vi "tap_stim_rec_async_2.vi"(0 "Convert Power to Voltage B":bool, 2 "voltages/power B":dbl[](array[numeric]), 3 "SSH password":string, 4 "Transfer and Run Date Folder After Experiment":bool, 5 "SSH user name":string, 6 "Tags":string, 7 "Frames":i32, 8 "Convert Power to Voltage":bool, 9 "voltages/power A":dbl[](array[numeric]), 10 "parameters":string[](array[string]), 11 "parameters headers":string[](array[string])) -> ()   [LabVIEW 2014]
uses:
  <vilib>/vision/driver/IMAQdx.llb/IMAQdx Acquisition Mode.ctl
  <vilib>/userdefined/High Color/IMAQdx.ctl
  <vilib>/vision/driver/IMAQdx.llb/IMAQdx Buffer Number Mode.ctl
  <vilib>/Utility/file.llb/Write To Spreadsheet File (DBL).vi
  <vilib>/Utility/file.llb/Write To Spreadsheet File (string).vi
  <vilib>/Utility/file.llb/Read From Spreadsheet File (string).vi
  <vilib>/vision/driver/NI_Vision_Acquisition_Software.lvlib
panel:
  out "Current Voltage B":dbl
  out "Current Voltage A":dbl
  out "Saved Buffer Number":u32
  out "ProcessFrameRate":dbl
  out "# elements in queue":i32
  out "CameraFrameRate":dbl
  out "Camera Buffer Number":u32
  out "Image":T1(plugin-control)
  out "JPEG Quality":dbl
  out "Error":string
  out "Save Directory":path
  in  "stop":bool
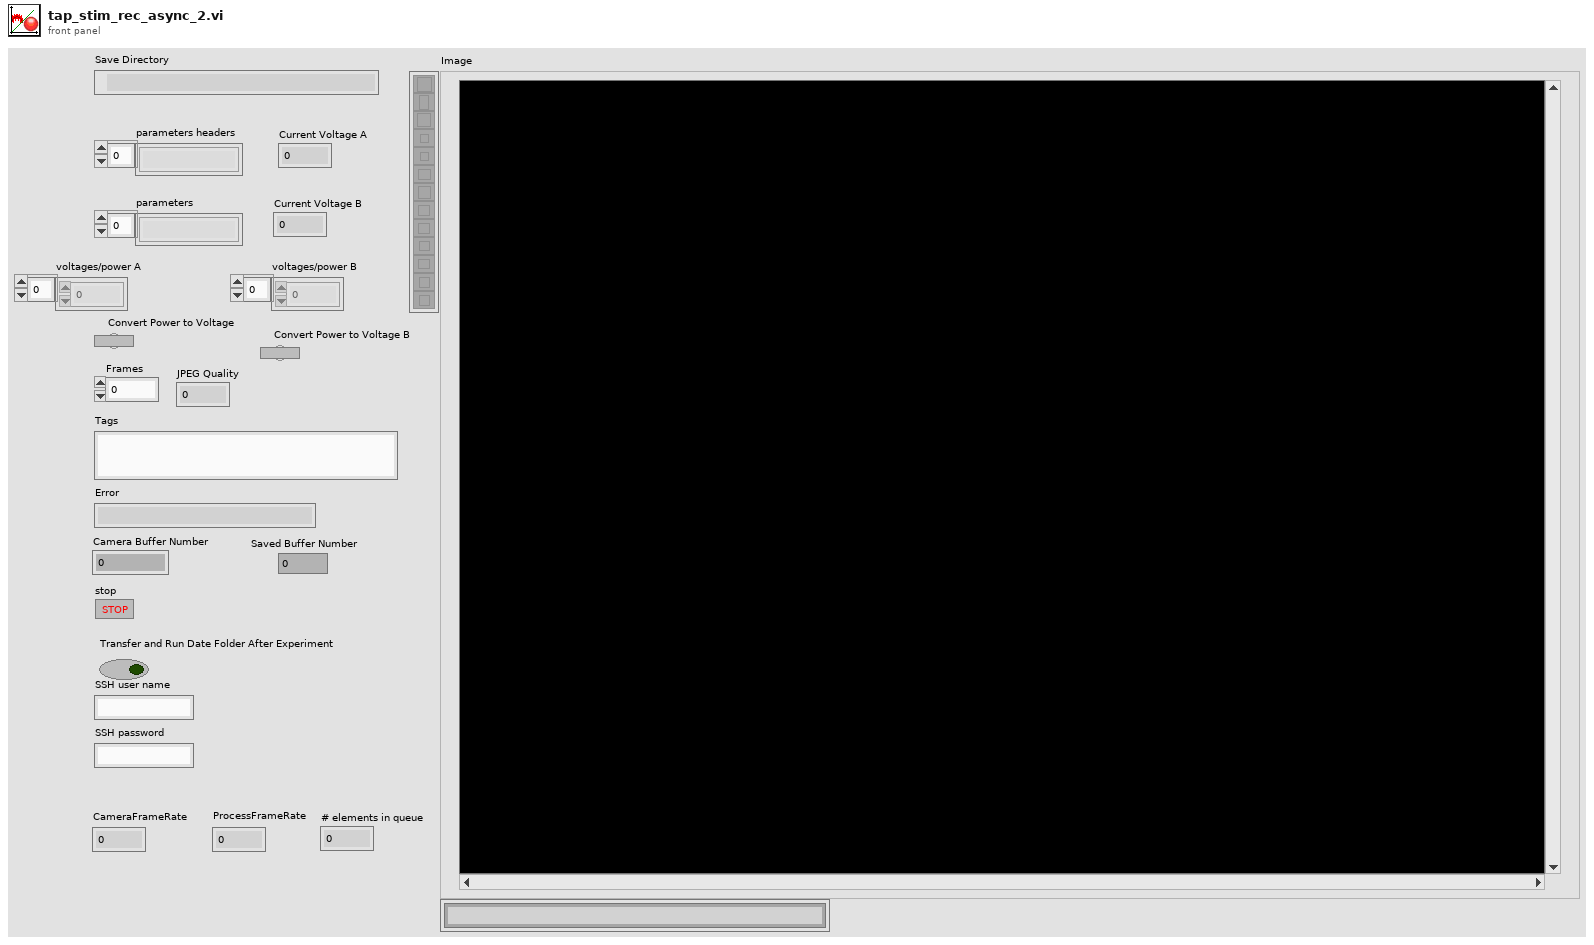
[diagram p1: front panel]
types:
  T1 = typedef "IMAQ Image.ctl" = refnum<image>
  T2 = typedef "IMAQdx.ctl" = refnum<k21>
  T3 = typedef "NI_Vision_Acquisition_Software.lvlib/IMAQdx Buffer Number Mode.ctl" = enum32{"Next", "Last", "Buffer Number"}
  T4 = typedef "Image Type" = u32
  T5 = typedef "NI_Vision_Acquisition_Software.lvlib/IMAQdx Acquisition Mode.ctl" = enum32{"One Shot", "Continuous"}
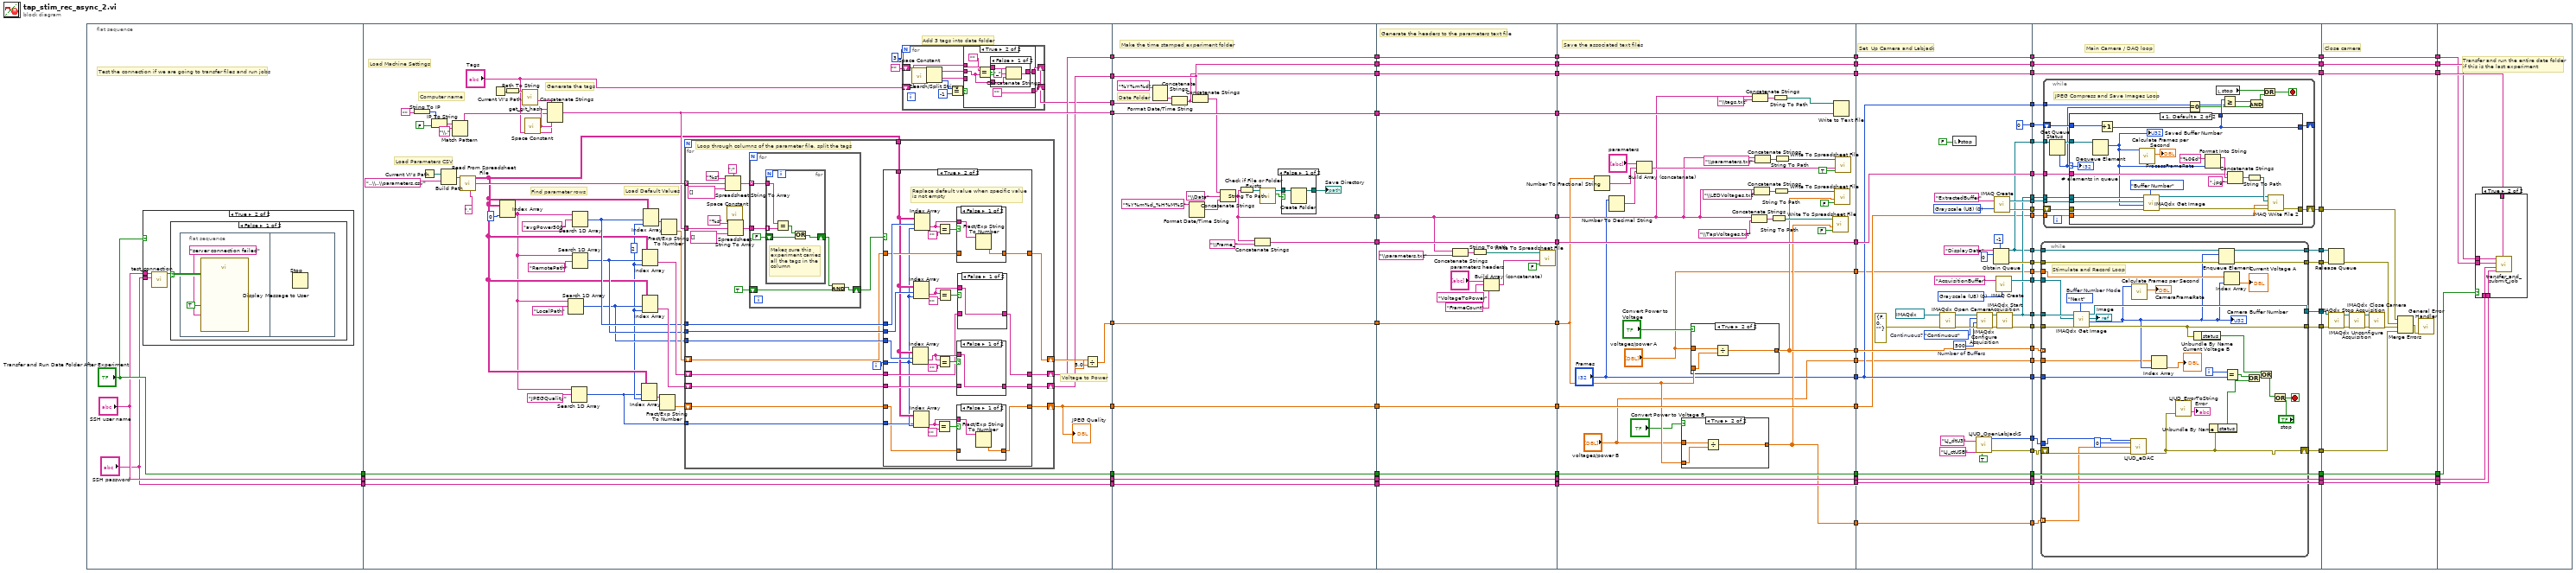
[diagram p0: block diagram]
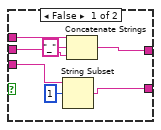
[diagram p4: hidden frame]
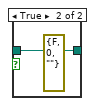
[diagram p11: hidden frame]
diagram:
  n1 = flat-sequence {
    tunnel: ["Transfer and Run Date Folder After Experiment"] -> w56
    tunnel: ["SSH user name"] -> w55
    tunnel: ["SSH password"] -> w54
    tunnel: [w138] -> w86
    tunnel: [w121] -> w85
    tunnel: [w112] -> w76
    tunnel: [w113] -> w75
    tunnel: w56 -> [w130]
    tunnel: w55 -> [w129]
    tunnel: w54 -> [w128]
    tunnel: [w130] -> w47
    tunnel: [w129] -> w40
    tunnel: [w128] -> w39
    tunnel: [w109] -> w32
    tunnel: [w100] -> w31
    tunnel: [w274] -> w70
    tunnel: [w273] -> w68
    tunnel: [w272] -> w66
    tunnel: [w271] -> w64
    tunnel: [w253] -> w62
    tunnel: [w255] -> w60
    tunnel: [w270] -> w58
    tunnel: w75 -> [w270]
    tunnel: w76 -> [w255]
    tunnel: w85 -> [w271]
    tunnel: w86 -> [w272]
    tunnel: [w262] -> w48
    tunnel: w47 -> [w262]
    tunnel: [w261] -> w41
    tunnel: w40 -> [w261]
    tunnel: w39 -> [w260]
    tunnel: [w260] -> w38
    tunnel: w32 -> [w256]
    tunnel: w31 -> [w252]
    tunnel: [w252] -> w28
    tunnel: w70 -> [w296]
    tunnel: [w296] -> w69
    tunnel: w68 -> [w282]
    tunnel: [w282] -> w67
    tunnel: w66 -> [w295]
    tunnel: [w295] -> w65
    tunnel: w64 -> [w294]
    tunnel: [w294] -> w63
    tunnel: w62 -> [w293]
    tunnel: [w293] -> w61
    tunnel: w60 -> [w292]
    tunnel: [w292] -> w59
    tunnel: w58 -> [w291]
    tunnel: [w291] -> w57
    tunnel: [w281] -> w49
    tunnel: w48 -> [w281]
    tunnel: [w280] -> w42
    tunnel: w41 -> [w280]
    tunnel: w38 -> [w279]
    tunnel: [w279] -> w37
    tunnel: [w278] -> w29
    tunnel: w28 -> [w278]
    tunnel: w69 -> [w331]
    tunnel: [w331] -> w91
    tunnel: [w301] -> w89
    tunnel: ["Frames"] -> w88
    tunnel: w67 -> [w302]
    tunnel: w65 -> [w308]
    tunnel: w63 -> [w311]
    tunnel: w61 -> [w320]
    tunnel: [w320] -> w81
    tunnel: [w319] -> w77
    tunnel: w59 -> [w319]
    tunnel: [w318] -> w71
    tunnel: w57 -> [w318]
    tunnel: [w314] -> w50
    tunnel: w49 -> [w314]
    tunnel: [w313] -> w43
    tunnel: w42 -> [w313]
    tunnel: w37 -> [w312]
    tunnel: [w312] -> w36
    tunnel: [w310] -> w30
    tunnel: w29 -> [w310]
    tunnel: [w300] -> w7
    tunnel: ["voltages/power A"] -> w6
    tunnel: ["voltages/power B"] -> w4
    tunnel: w91 -> [w352]
    tunnel: [w380] -> w90
    tunnel: w89 -> [w380]
    tunnel: w88 -> [w351]
    tunnel: [w351] -> w87
    tunnel: [w379] -> w82
    tunnel: w81 -> [w379]
    tunnel: [w378] -> w78
    tunnel: w77 -> [w378]
    tunnel: [w377] -> w72
    tunnel: w71 -> [w377]
    tunnel: [w376] -> w51
    tunnel: w50 -> [w376]
    tunnel: [w375] -> w44
    tunnel: w43 -> [w375]
    tunnel: w36 -> [w374]
    tunnel: [w374] -> w35
    tunnel: w30 -> [w349]
    tunnel: [w358] -> w27
    tunnel: [w353] -> w26
    tunnel: [w357] -> w25
    tunnel: [w356] -> w24
    tunnel: [w350] -> w23
    tunnel: [w355] -> w20
    tunnel: [w354] -> w19
    tunnel: [w353] -> w18
    tunnel: [w352] -> w17
    tunnel: [w351] -> w16
    tunnel: [w350] -> w15
    tunnel: [w349] -> w14
    tunnel: [0] -> w10
    tunnel: [w346] -> w8
    tunnel: w7 -> [w346]
    tunnel: w6 -> [w345]
    tunnel: [w345] -> w5
    tunnel: w4 -> [w344]
    tunnel: [w344] -> w3
    tunnel: [w343] -> w2
    tunnel: [w342] -> w1
    tunnel: w90 -> [w398]
    tunnel: w87 -> [w399]
    tunnel: [w415] -> w83
    tunnel: w82 -> [w415]
    tunnel: [w414] -> w79
    tunnel: w78 -> [w414]
    tunnel: [w413] -> w73
    tunnel: w72 -> [w413]
    tunnel: [w412] -> w52
    tunnel: w51 -> [w412]
    tunnel: [w411] -> w45
    tunnel: w44 -> [w411]
    tunnel: w35 -> [w410]
    tunnel: [w410] -> w34
    tunnel: w27 -> [w393]
    tunnel: w26 -> [w394]
    tunnel: w25 -> [w395]
    tunnel: w24 -> [w396]
    tunnel: w23 -> [w397]
    tunnel: [w389] -> w22
    tunnel: [w388] -> w21
    tunnel: w20 -> [w409]
    tunnel: w19 -> [w408]
    tunnel: w18 -> [w407]
    tunnel: w17 -> [w406]
    tunnel: w16 -> [w405]
    tunnel: w15 -> [w404]
    tunnel: w14 -> [w403]
    tunnel: [w387] -> w13
    tunnel: [w390] -> w12
    tunnel: [w402] -> w11
    tunnel: w10 -> [w401]
    tunnel: [w391] -> w9
    tunnel: w8 -> [w392]
    tunnel: w5 -> [w386]
    tunnel: w3 -> [w385]
    tunnel: w2 -> [w400]
    tunnel: w1 -> [w384]
    tunnel: [w505] -> w84
    tunnel: w83 -> [w505]
    tunnel: [w504] -> w80
    tunnel: w79 -> [w504]
    tunnel: [w503] -> w74
    tunnel: w73 -> [w503]
    tunnel: [w502] -> w53
    tunnel: w52 -> [w502]
    tunnel: [w501] -> w46
    tunnel: w45 -> [w501]
    tunnel: w34 -> [w500]
    tunnel: [w500] -> w33
    tunnel: w22 -> [w495]
    tunnel: w21 -> [w494]
    tunnel: w13 -> [w489]
    tunnel: w12 -> [w492]
    tunnel: w11 -> [w491]
    tunnel: w9 -> [w490]
    tunnel: w84 -> [w511]
    tunnel: w80 -> [w510]
    tunnel: w74 -> [w509]
    tunnel: w53 -> [w508]
    tunnel: w46 -> [w507]
    tunnel: w33 -> [w506]
    frame #0 {
      # "Test the connection if we are going to transfer files and run jobs"
      n2 = case shown="True" "Transfer and Run Date Folder After Experiment" {
        tunnel: "SSH password" -> [_ w97]
        tunnel: "SSH user name" -> [_ w95]
        frame False {
        }
        frame True {
          n3 = call "test_connection.vi"("Username"=w95, "Password"=w97) -> ("Connection Successful"=w96:bool)  [unwired: 7 in]
          n4 = case shown="False" w96 {
            frame False {
              n5 = flat-sequence {
                frame #0 {
                  n6 = call "Display Message to User"("Enable"=TRUE, "Message"="server connection failed") -> ()  [unwired: 8 in, 2 out]
                }
                frame #1 {
                  n7 = Stop() -> ()  [unwired: 1 in]
                }
              }
            }
            frame True {
            }
          }
        }
      }
    }
    frame #1 {
      w103 = 2
      # "Add 3 tags into date folder"
      # "Generate the tags"
      # "Find parameter rows"
      # "Load Default Values"
      # "Voltage to Power"
      # "Load Parameters CSV"
      # "Computer name"
      # "Load Machine Settings"
      n8 = String To IP(1:"") -> (0:w146:u32)
      n9 = Current VI's Path() -> (path=w141:path)
      n10 = IP To String(1:FALSE, 2:w146) -> (0:w143:string)
      n11 = Build Path(base path=w141, name or relative path="..\\..\\parameters.csv") -> (appended path=w132:path)
      n12 = Match Pattern(string=w143, regular expression="\\.") -> (before substring=w123:string)  [unwired: 1 in, 3 out]
      n13 = call-poly <vilib>:"Read From Spreadsheet File.vi"("delimiter (\\t)"=",", "file path (dialog if empty)"=w132) -> ("first row"=w122:string[], "all rows"=w105:string[][])  [unwired: 5 in, 3 out]
      n14 = Current VI's Path() -> (path=w125:path)
      n15 = Index Array(array=w105, index (col)=0) -> (element=w104:string[])  [unwired: 1 in]
      n16 = Path To String(path=w125) -> (string=w124:string)
      n17 = call "get_git_hash.vi"("VI folder"=w124) -> ("github hash"=w127:string)  [unwired: 10 in]
      n18 = call <vilib>:"Space Constant.vi"() -> ("String"=w126:string)
      n19 = Concatenate Strings(w127, w126, w123, w126, "Tags") -> (w121:string)
      n20 = Search 1D Array(1D array=w104, element="LocalPath") -> (index of element=w115:i32)  [unwired: 1 in]
      n21 = Search 1D Array(1D array=w104, element="JPEGQuality") -> (index of element=w101:i32)  [unwired: 1 in]
      n22 = Search 1D Array(1D array=w104, element="RemotePath") -> (index of element=w116:i32)  [unwired: 1 in]
      n23 = Search 1D Array(1D array=w104, element="avgPower500") -> (index of element=w117:i32)  [unwired: 1 in]
      n24 = Index Array(array=w105, index (row)=w101, index (col)=w103) -> (element=w106:string)
      n25 = Index Array(array=w105, index (row)=w116, index (col)=w103) -> (element=w119:string)
      n26 = Index Array(array=w105, index (row)=w115, index (col)=w103) -> (element=w118:string)
      n27 = Index Array(array=w105, index (row)=w117, index (col)=w103) -> (element=w134:string)
      n28 = Fract/Exp String To Number(string=w106) -> (number=w102:dbl)  [unwired: 3 in, 1 out]
      n29 = Fract/Exp String To Number(string=w134) -> (number=w120:dbl)  [unwired: 3 in, 1 out]
      n30 = for {
        tunnel: w122 -> [w200] mode=indexing
        tunnel: w121 -> [w192]
        tunnel: w117 -> [w187]
        tunnel: w116 -> [w186]
        tunnel: w115 -> [w185]
        tunnel: w105 -> [w190]
        shift-right: [w182] -> w114
        shift-left: w120 -> [w183]
        shift-right: [w179] -> w113
        shift-left: w119 -> [w180]
        shift-right: [w178] -> w112
        shift-left: w118 -> [w181]
        shift-right: [w175] -> w100
        shift-left: w102 -> [w177]
        tunnel: w101 -> [w176]
        i -> [w184]
        # "Loop through columns of the parameter file, split the tags"
        n31 = Spreadsheet String To Array(delimiter (Tab)=";", format string="%s", spreadsheet string=w200, array type (2D Dbl)=string[] []) -> (array=w196:string[])
        n32 = call <vilib>:"Space Constant.vi"() -> ("String"=w194:string)
        n33 = Spreadsheet String To Array(delimiter (Tab)=w194, format string="%s", spreadsheet string=w192, array type (2D Dbl)=string[] []) -> (array=w191:string[])
        n34 = for {
          tunnel: w196 -> [w246] mode=indexing
          tunnel: w191 -> [w245]
          shift-right: [w243] -> w188
          shift-left: TRUE -> [w241]
          n35 = for {
            tunnel: w246 -> [w251]
            tunnel: w245 -> [w250] mode=indexing
            shift-right: [w247] -> w242
            shift-left: FALSE -> [w248]
            # "Makes sure this\nexperiment carries\nall the tags in the\ncolumn"
            n36 = Equal?(x=w251, y=w250) -> (x = y?=w249:bool)
            n37 = Or(x=w249, y=w248) -> (x .or. y?=w247:bool)
          }
          n38 = And(x=w242, y=w241) -> (x .and. y?=w243:bool)
        }
        n39 = case shown="True" w188 {
          tunnel: w183 -> [w204 w225]
          tunnel: [w204 w224] -> w182
          tunnel: w187 -> [_ w230]
          tunnel: w186 -> [_ w229]
          tunnel: w185 -> [_ w228]
          tunnel: w184 -> [_ w207]
          tunnel: w190 -> [_ w208]
          tunnel: [w203 w214] -> w179
          tunnel: [w202 w216] -> w178
          tunnel: w181 -> [w202 w215]
          tunnel: w180 -> [w203 w213]
          tunnel: w177 -> [w201 w205]
          tunnel: w176 -> [_ w206]
          tunnel: [w201 w209] -> w175
          frame False {
          }
          frame True {
            # "Replace default value when specific value\nis not empty"
            n40 = Index Array(array=w208, index (row)=w228, index (col)=w207) -> (element=w217:string)
            n41 = Index Array(array=w208, index (row)=w229, index (col)=w207) -> (element=w220:string)
            n42 = Index Array(array=w208, index (row)=w206, index (col)=w207) -> (element=w210:string)
            n43 = Index Array(array=w208, index (row)=w230, index (col)=w207) -> (element=w223:string)
            n44 = Equal?(x=w210, y="") -> (x = y?=w211:bool)
            n45 = Equal?(x=w223, y="") -> (x = y?=w226:bool)
            n46 = Equal?(x=w217, y="") -> (x = y?=w218:bool)
            n47 = Equal?(x=w220, y="") -> (x = y?=w221:bool)
            n48 = case shown="False" w211 {
              tunnel: w205 -> [_ w233]
              tunnel: [w232 w233] -> w209
              tunnel: w210 -> [w231 _]
              frame False {
                n49 = Fract/Exp String To Number(string=w231) -> (number=w232:dbl)  [unwired: 3 in, 1 out]
              }
              frame True {
              }
            }
            n50 = case shown="False" w226 {
              tunnel: w225 -> [_ w240]
              tunnel: [w239 w240] -> w224
              tunnel: w223 -> [w238 _]
              frame False {
                n51 = Fract/Exp String To Number(string=w238) -> (number=w239:dbl)  [unwired: 3 in, 1 out]
              }
              frame True {
              }
            }
            n52 = case shown="False" w218 {
              tunnel: w217 -> [w234 _]
              tunnel: [w234 w235] -> w216
              tunnel: w215 -> [_ w235]
              frame False {
              }
              frame True {
              }
            }
            n53 = case shown="False" w221 {
              tunnel: w220 -> [w236 _]
              tunnel: [w236 w237] -> w214
              tunnel: w213 -> [_ w237]
              frame False {
              }
              frame True {
              }
            }
          }
        }
      }
      "JPEG Quality" <- w100
      n54 = for {
        N: 3 -> [_]
        shift-right: [w147] -> _
        shift-left: "Tags" -> [w156]
        shift-right: [w149] -> w109
        shift-left: "" -> [w154]
        n55 = call <vilib>:"Space Constant.vi"() -> ("String"=w155:string)
        n56 = Search/Split String(string=w156, search string/char (-)=w155) -> (substring before match=w153:string, match + rest of string=w152:string, offset of match=w151:i32)  [unwired: 1 in]
        n57 = Equal?(x=w151, y=-1) -> (x = y?=w148:bool)
        n58 = case shown="True" w148 {
          tunnel: w154 -> [w157 w167]
          tunnel: w153 -> [w158 w164]
          tunnel: w152 -> [w159 _]
          tunnel: [w161 ""] -> w147
          tunnel: [w160 w166] -> w149
          frame False {
            n59 = String Subset(string=w159, offset (0)=1) -> (substring=w161:string)  [unwired: 1 in]
            n60 = Concatenate Strings(w157, "_", w158) -> (w160:string)
          }
          frame True {
            n61 = Equal?(x="", y=w164) -> (x = y?=w168:bool)
            n62 = case shown="False" w168 {
              tunnel: w167 -> [w171 w174]
              tunnel: [w172 w174] -> w166
              tunnel: w164 -> [w170 _]
              frame False {
                n63 = Concatenate Strings(w171, "_", w170) -> (w172:string)
              }
              frame True {
              }
            }
          }
        }
      }
      n64 = Divide(x=w114, y=5.0) -> (x/y=w138:dbl)
    }
    frame #2 {
      # "Make the time stamped experiment folder"
      # "Date Folder"
      n65 = Format Date/Time String(time format string (%c)="%Y%m%d") -> (date/time string=w257:string)  [unwired: 2 in]
      n66 = Concatenate Strings(w257, w256) -> (w253:string)
      n67 = Format Date/Time String(time format string (%c)="%Y%m%d_%H%M%S") -> (date/time string=w259:string)  [unwired: 2 in]
      n68 = Concatenate Strings(w255, w253) -> (w254:string)
      n69 = Concatenate Strings(w254, "\\Data", w259) -> (w273:string)
      n70 = String To Path(string=w273) -> (path=w265:path)
      n71 = Concatenate Strings(w273, "\\Frame_") -> (w274:string)
      n72 = call <vilib>:"Check if File or Folder Exists.vi"("path"=w265) -> ("file or folder exists?"=w268:bool, "dup path"=w267:path)  [unwired: 8 in, 1 out]
      n73 = case shown="False" w268 {
        tunnel: [w275 w277] -> w264
        tunnel: w267 -> [w276 w277]
        frame False {
          n74 = Create Folder(path (use dialog)=w276) -> (created path=w275:path)  [unwired: 2 in, 2 out]
        }
        frame True {
          (unwired) errorcluster {"status"=FALSE, "code"=0, "source"=""} ("error out")
        }
      }
      "Save Directory" <- w264
    }
    frame #3 {
      # "Generate the headers to the parameters text file"
      n75 = Concatenate Strings(w282, "\\parameters.txt") -> (w290:string)
      n76 = String To Path(string=w290) -> (path=w289:path)
      n77 = Build Array (concatenate)("parameters headers", "VoltageToPower", "FrameCount") -> (w286:string[])
      n78 = call-poly <vilib>:"Write To Spreadsheet File.vi"("append to file? (new file:F)"=FALSE, "1D data"=w286, "file path (dialog if empty)"=w289) -> ()  [unwired: 5 in, 1 out]
    }
    frame #4 {
      # "Save the associated text files"
      n79 = Number To Fractional String(number=w308) -> (F-format string=w315:string)  [unwired: 3 in]
      n80 = Number To Decimal String(number="Frames") -> (decimal integer string=w316:string)  [unwired: 1 in]
      n81 = Build Array (concatenate)("parameters", w315, w316) -> (w324:string[])
      n82 = case shown="True" "Convert Power to Voltage B" {
        tunnel: "voltages/power B" -> [w334 w337]
        tunnel: [w334 w335] -> w300
        tunnel: w308 -> [_ w336]
        frame False {
        }
        frame True {
          n83 = Divide(x=w337, y=w336) -> (x/y=w335:dbl[])
        }
      }
      n84 = case shown="True" "Convert Power to Voltage" {
        tunnel: "voltages/power A" -> [w338 w341]
        tunnel: [w338 w339] -> w301
        tunnel: w308 -> [_ w340]
        frame False {
        }
        frame True {
          n85 = Divide(x=w341, y=w340) -> (x/y=w339:dbl[])
        }
      }
      n86 = Concatenate Strings(w302, "\\TapVoltages.txt") -> (w306:string)
      n87 = Concatenate Strings(w302, "\\tags.txt") -> (w322:string)
      n88 = Concatenate Strings(w302, "\\LEDVoltages.txt") -> (w333:string)
      n89 = Concatenate Strings(w302, "\\parameters.txt") -> (w328:string)
      n90 = String To Path(string=w306) -> (path=w305:path)
      n91 = String To Path(string=w322) -> (path=w321:path)
      n92 = String To Path(string=w333) -> (path=w332:path)
      n93 = String To Path(string=w328) -> (path=w327:path)
      n94 = call-poly <vilib>:"Write To Spreadsheet File.vi"("append to file? (new file:F)"=FALSE, "1D data"=w300, "file path (dialog if empty)"=w305) -> ()  [unwired: 5 in, 1 out]
      n95 = Write to Text File(file (use dialog)=w321, text=w311) -> ()  [unwired: 2 in, 3 out]
      n96 = call-poly <vilib>:"Write To Spreadsheet File.vi"("append to file? (new file:F)"=FALSE, "1D data"=w301, "file path (dialog if empty)"=w332) -> ()  [unwired: 5 in, 1 out]
      n97 = call-poly <vilib>:"Write To Spreadsheet File.vi"("append to file? (new file:F)"=TRUE, "1D data"=w324, "file path (dialog if empty)"=w327) -> ()  [unwired: 5 in, 1 out]
    }
    frame #5 {
      w361 = T4 0 items=["Grayscale (U8)", "Grayscale (I16)", "Grayscale (SGL)", "Complex (CSG)", "RGB (U32)", "HSL (U32)", "RGB (U64)"] ("Image Type")
      w370 = T4 0 items=["Grayscale (U8)", "Grayscale (I16)", "Grayscale (SGL)", "Complex (CSG)", "RGB (U32)", "HSL (U32)", "RGB (U64)"] ("Image Type")
      w371 = u32 500  # Number of Buffers
      w367 = IMAQdx_Acquisition_Mode."Continuous"  # Continuous?
      # "Set  Up Camera and Labjack"
      n98 = call <vilib>:"IMAQdx Open Camera.vi"("error in"=errorcluster {"status"=FALSE, "code"=0, "source"=""}, "Session In"=T2 "cam0") -> ("error out"=w372:errorcluster, "Session Out"=w373:T2)  [unwired: 8 in]
      n99 = local write "stop"(FALSE) -> ()
      n100 = call "LJUD_OpenLabJackS.vi"("FirstFound"=TRUE, "ConnectionType"="LJ_ctUSB", "DeviceType"="LJ_dtU3") -> ("error out"=w342:errorcluster, "Handle"=w343:i32)  [unwired: 6 in, 1 out]
      n101 = call <vilib>:"IMAQdx Configure Acquisition.vi"("error in"=w372, "Number of Buffers"=w371, "Continuous?"=w367, "Session In"=w373) -> ("error out"=w368:errorcluster, "Session Out"=w366:T2)  [unwired: 6 in]
      n102 = Obtain Queue(max queue size (-1, unlimited)=-1, name (unnamed)="DisplayData", element data type=u32 0) -> (queue out=w350:refnum<queue>, error out=w356:errorcluster)  [unwired: 2 in, 1 out]
      n103 = call "IMAQ Create"("Image Name"="ExtractedBuffer", "Image Type"=w361) -> ("New Image"=w354:T1, "error out"=w355:errorcluster)  [unwired: 3 in]
      n104 = call "IMAQ Create"("Image Name"="AcquisitionBuffer", "Image Type"=w370) -> ("New Image"=w357:T1)  [unwired: 3 in, 1 out]
      n105 = call <vilib>:"IMAQdx Start Acquisition.vi"("error in"=w368, "Session In"=w366) -> ("error out"=w358:errorcluster, "Session Out"=w353:T2)  [unwired: 8 in]
    }
    frame #6 {
      # "Main Camera / DAQ loop"
      n106 = while {
        shift-right: [w418] -> w387
        shift-left: w384 -> [w420]
        tunnel: w398 -> [_] mode=indexing
        tunnel: w399 -> [w442]
        tunnel: w393 -> [w438]
        tunnel: w394 -> [w437]
        tunnel: w395 -> [w436]
        tunnel: w396 -> [w435]
        tunnel: w397 -> [w434]
        tunnel: [w430] -> w391
        tunnel: [w429] -> w390
        tunnel: [w428] -> w389
        tunnel: [w427] -> w388
        tunnel: w400 -> [w421]
        tunnel: w392 -> [w416] mode=indexing
        tunnel: w386 -> [w425]
        tunnel: w385 -> [w422]
        i -> [w443]
        stop <- w447 stop-if-true
        w441 = IMAQdx_Buffer_Number_Mode."Next"  # Buffer Number Mode
        # "Stimulate and Record Loop"
        n107 = call <vilib>:"IMAQdx Get Image.vi"("Buffer Number Mode (Next)"=w441, "error in"=w438, "Image In"=w436, "Session In"=w437) -> ("error out"=w427:errorcluster, "Buffer Number Out"=w423:u32, "Image Out"=→"Image":T1, "Session Out"=w428:T2)  [unwired: 4 in]
        "Camera Buffer Number" <- w423
        n108 = call "LJUD_eDAC.vi"("Handle In"=w421, "Channel"=0, "Voltage"=w416, "error in"=w420) -> ("error out"=w418:errorcluster)  [unwired: 10 in, 1 out]
        n109 = call <vilib>:"Calculate Frames per Second.vi"("Buffer Number"=w423) -> ("Processed Frames/s"=→"CameraFrameRate":dbl)  [unwired: 8 in, 2 out]
        n110 = Index Array(array=w422, index=w423) -> (element=→"Current Voltage B":dbl)
        n111 = call "LJUD_ErrorToString.vi"("error in"=w418) -> ("String"=→"Error":string)  [unwired: 10 in]
        n112 = Unbundle By Name(w427) -> ("status"=w433:bool)
        n113 = Unbundle By Name(w418) -> ("status"=w417:bool)
        n114 = Enqueue Element(queue=w434, element=w423, error in (no error)=w435) -> (queue out=w430:refnum<queue>, error out=w429:errorcluster)  [unwired: 1 in, 1 out]
        n115 = Index Array(array=w425, index=w423) -> (element=→"Current Voltage A":dbl)
        n116 = Equal?(x=w443, y=w442) -> (x = y?=w444:bool)
        n117 = Or(x=w444, y=w417) -> (x .or. y?=w432:bool)
        n118 = Or(x=w433, y=w432) -> (x .or. y?=w431:bool)
        n119 = Or(x=w431, y="stop") -> (x .or. y?=w447:bool)
      }
      n120 = while {
        tunnel: w404 -> [w465]
        tunnel: w408 -> [w463]
        tunnel: w407 -> [w462]
        tunnel: w406 -> [w460]
        shift-right: [w459] -> w402
        shift-left: w409 -> [w461]
        tunnel: w405 -> [w452]
        tunnel: w403 -> [w457]
        shift-right: [w454] -> _
        shift-left: w401 -> [w455]
        stop <- w458 stop-if-true
        # "JPEG Compress and Save Images Loop"
        n121 = Get Queue Status(queue=w465) -> (queue out=w464:refnum<queue>, # elements in queue=w448:i32)  [unwired: 2 in, 6 out]
        n122 = case shown="1, Default" w448 {
          selector: w448 -> [_ w486]
          tunnel: w464 -> [_ w484]
          tunnel: w463 -> [_ w483]
          tunnel: w462 -> [_ w482]
          tunnel: w461 -> [w467 w481]
          tunnel: w460 -> [_ w475]
          tunnel: [w467 w471] -> w459
          tunnel: w457 -> [_ w470]
          tunnel: w455 -> [w466 w469]
          tunnel: [w466 w468] -> w454
          tunnel: [w466 w468] -> w453
          frame 0 {
          }
          frame 1, Default {
            n123 = Dequeue Element(queue=w484) -> (element=w472:u32)  [unwired: 2 in, 3 out]
            "Saved Buffer Number" <- w472
            n124 = Increment(x=w469) -> (x+1=w468:i32)
            n125 = call <vilib>:"Calculate Frames per Second.vi"("Buffer Number"=w472) -> ("Processed Frames/s"=→"ProcessFrameRate":dbl)  [unwired: 8 in, 2 out]
            n126 = call <vilib>:"IMAQdx Get Image.vi"("Buffer Number Mode (Next)"=IMAQdx_Buffer_Number_Mode."Buffer Number", "error in"=w481, "Buffer Number In"=w472, "Image In"=w483, "Session In"=w482) -> ("error out"=w473:errorcluster, "Image Out"=w474:T1)  [unwired: 3 in, 2 out]
            n127 = Format Into String(format string="%06d" ("string"), w472) -> (resulting string=w477:string)  [unwired: 2 in, 1 out]
            n128 = Concatenate Strings(w475, w477, ".jpg" ("string")) -> (w479:string)
            n129 = String To Path(string=w479) -> (path=w478:path)
            n130 = call-poly "IMAQ Write File 2"("error in (no error)"=w473, "Image Quality"=w470, "File Path"=w478, "Image"=w474) -> ("error out"=w471:errorcluster)  [unwired: 6 in, 1 out]
            "# elements in queue" <- w486
          }
        }
        n131 = Equal To 0?(x=w448) -> (x = 0?=w449:bool)
        n132 = local read "stop"() -> (w456:bool)
        n133 = Greater Or Equal?(x=w453, y=w452) -> (x >= y?=w451:bool)
        n134 = And(x=w451, y=w449) -> (x .and. y?=w450:bool)
        n135 = Or(x=w456, y=w450) -> (x .or. y?=w458:bool)
      }
    }
    frame #7 {
      # "Close camera"
      n136 = Release Queue(queue=w490) -> ()  [unwired: 2 in, 3 out]
      n137 = call <vilib>:"IMAQdx Stop Acquisition.vi"("error in"=w494, "Session In"=w495) -> ("error out"=w496:errorcluster, "Session Out"=w497:T2)  [unwired: 8 in]
      n138 = call <vilib>:"IMAQdx Unconfigure Acquisition.vi"("error in"=w496, "Session In"=w497) -> ("error out"=w499:errorcluster, "Session Out"=w498:T2)  [unwired: 8 in]
      n139 = call <vilib>:"IMAQdx Close Camera.vi"("error in"=w499, "Session In"=w498) -> ("error out"=w488:errorcluster)  [unwired: 9 in]
      n140 = Merge Errors(w491, w492, w488, w489) -> (w493:errorcluster)
      n141 = call <vilib>:"General Error Handler.vi"("error in (no error)"=w493) -> ()  [unwired: 10 in, 5 out]
    }
    frame #8 {
      # "Transfer and run the entire date folder\nif this is the last experiment"
      n142 = case shown="True" w508 {
        tunnel: w511 -> [_ w516]
        tunnel: w510 -> [_ w515]
        tunnel: w509 -> [_ w514]
        tunnel: w507 -> [_ w513]
        tunnel: w506 -> [_ w512]
        frame False {
        }
        frame True {
          n143 = call "transfer_and_submit_job.vi"("Date Folder"=w516, "Password"=w512, "Username"=w513, "Remote Data Directory"=w514, "Local Data Directory"=w515) -> ()  [unwired: 7 in]
        }
      }
    }
  }
